vi "ADO Command Set Command Text.vi"(8 "error in (no error)":errorcluster, 10 "CommandText":string, 11 "ADODB._Command In":refnum<k7>) -> (0 "error out":errorcluster, 3 "ADODB._Command Out":refnum<k7>)   [LabVIEW 2013]
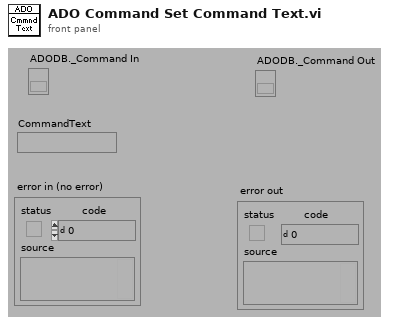
[diagram p1: front panel]
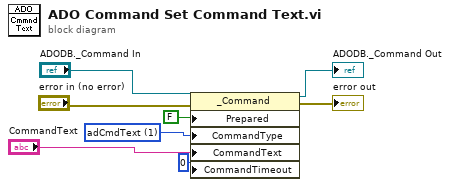
[diagram p0: block diagram]
diagram:
  w3 = 1 items=["adCmdUnspecified"=-1, "adCmdUnknown"=8, "adCmdText"=1, "adCmdTable"=2, "adCmdStoredProc"=4, "adCmdFile"=256, "adCmdTableDirect"=512] ("CommandType")
  n1 = property class="_Command"(reference="ADODB._Command In", error in="error in (no error)", "Prepared"=FALSE, "CommandType"=w3, "CommandText"="CommandText", "CommandTimeout"=0) -> (reference out=→"ADODB._Command Out":refnum<k7>, error out=→"error out":errorcluster)
